vi "send.vi"(8 "error in (no error)":errorcluster, 10 "messge":string, 11 "TCP_IP (in)":refnum<class "TCP_IP.lvclass">) -> (0 "error out":errorcluster, 3 "TCP_IP":refnum<class "TCP_IP.lvclass">)   [LabVIEW 2013, in "TCP_IP.lvclass"]
uses:
  TCP_IP.lvclass
  TCP_IP.lvclass/TCP_IP.ctl
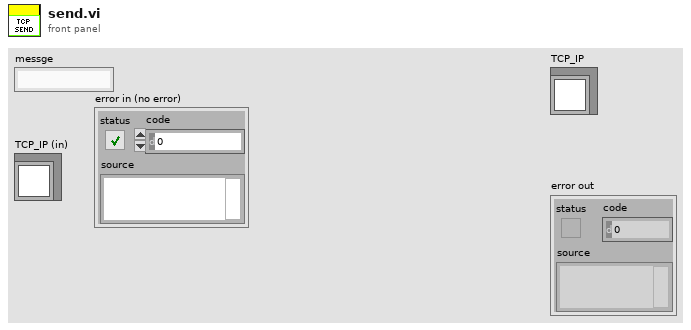
[diagram p1: front panel]
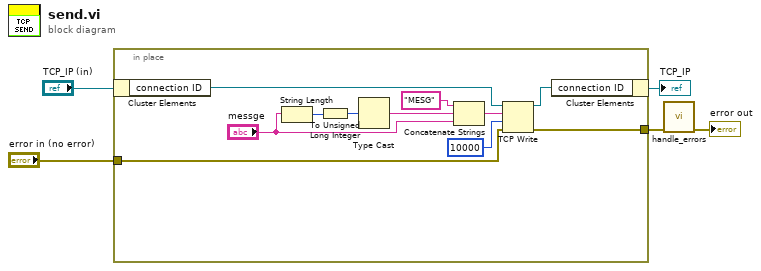
[diagram p0: block diagram]
diagram:
  n1 = in-place {
    in-place-border: [w7] -> w3
    in-place-border: "error in (no error)" -> [w6]
    n2 = in-place-cluster #1("TCP_IP (in)") -> ("connection ID"=w9:refnum<k5>)
    n3 = String Length(string="messge") -> (length=w12:i32)
    n4 = To Unsigned Long Integer(number=w12) -> (unsigned 32bit integer=w15:u32)
    n5 = Type Cast(x=w15) -> (*(type *) &x=w14:string)  [unwired: 1 in]
    n6 = Concatenate Strings("MESG", w14, "messge") -> (w11:string)
    n7 = TCP Write(connection ID=w9, data in=w11, error in (no error)=w6, 9:10000 ("timeout ms (25000)")) -> (connection ID out=w8:refnum<k5>, error out=w7:errorcluster)  [unwired: 1 out]
    n8 = in-place-cluster #1("connection ID"=w8) -> (→"TCP_IP":refnum<class "TCP_IP.lvclass">)
  }
  n9 = call "handle_errors.vi"("error in (no error)"=w3) -> ("error out"=→"error out":errorcluster)  [unwired: 10 in]
